vi "Configure Measurement Limits.vi"(7 "Upper Limit (2.0000000E+0)":dbl=2.0 format="%.7e", 8 "error in (no error)":errorcluster, 9 "Lower Limit (2.0000000E+0)":dbl=2.0 format="%.7e", 10 "Measurement Function (0: Voltage)":i32(ring) items=["Voltage", "Current", "Resistance"], 11 "VISA resource name":refnum<visa-resource-name>) -> (0 "error out":errorcluster, 3 "VISA resource name out":refnum<visa-resource-name>)   [LabVIEW 2019, in "Keithley 6517.lvlib"]
doc: "Configures the lower and upper limits for the measurement functions (Voltage, Current, Resistance and Charge).\n\nNote:\nThe specified measurement should be enabled from <b>Configure Measurement Function.vi</b>."
uses:
  Keithley 6517.lvlib
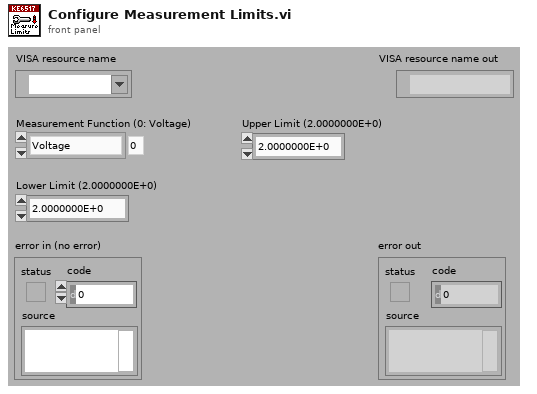
[diagram p1: front panel]
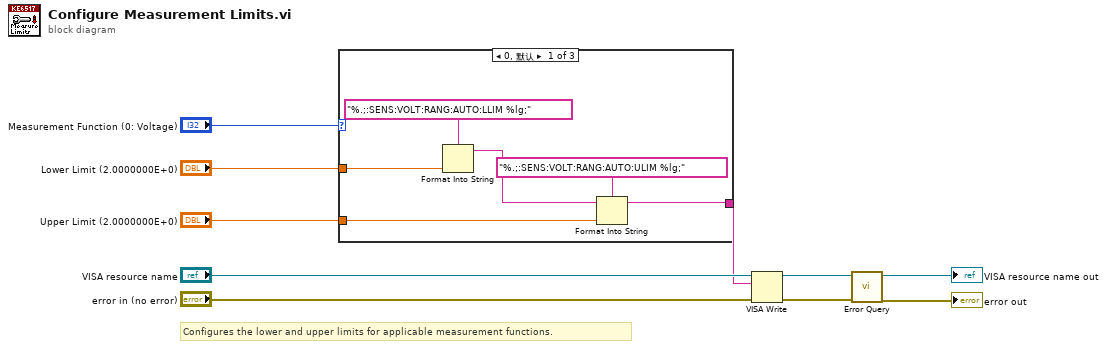
[diagram p0: block diagram]
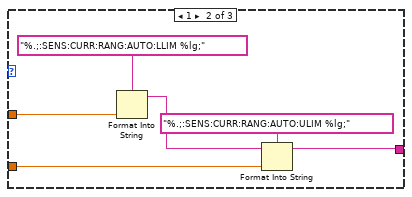
[diagram p2: hidden frame]
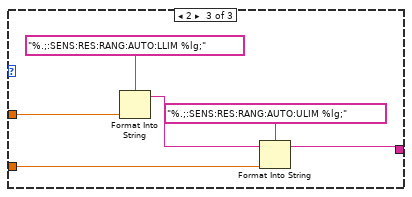
[diagram p3: hidden frame]
diagram:
  # "Configures the lower and upper limits for applicable measurement functions."
  n1 = case shown="0, 默认" "Measurement Function (0: Voltage)" {
    tunnel: "Lower Limit (2.0000000E+0)" -> [w13 w19 w25]
    tunnel: "Upper Limit (2.0000000E+0)" -> [w12 w18 w24]
    tunnel: [w11 w17 w23] -> w2
    frame 0, Default {
      n2 = Format Into String(format string="%.;:SENS:VOLT:RANG:AUTO:LLIM %lg;", w13) -> (resulting string=w15:string)  [unwired: 2 in, 1 out]
      n3 = Format Into String(format string="%.;:SENS:VOLT:RANG:AUTO:ULIM %lg;", initial string=w15, w12) -> (resulting string=w11:string)  [unwired: 1 in, 1 out]
    }
    frame 1 {
      n4 = Format Into String(format string="%.;:SENS:CURR:RANG:AUTO:LLIM %lg;", w19) -> (resulting string=w21:string)  [unwired: 2 in, 1 out]
      n5 = Format Into String(format string="%.;:SENS:CURR:RANG:AUTO:ULIM %lg;", initial string=w21, w18) -> (resulting string=w17:string)  [unwired: 1 in, 1 out]
    }
    frame 2 {
      n6 = Format Into String(format string="%.;:SENS:RES:RANG:AUTO:LLIM %lg;", w25) -> (resulting string=w28:string)  [unwired: 2 in, 1 out]
      n7 = Format Into String(format string="%.;:SENS:RES:RANG:AUTO:ULIM %lg;", initial string=w28, w24) -> (resulting string=w23:string)  [unwired: 1 in, 1 out]
    }
  }
  n8 = VISA Write(VISA resource name="VISA resource name", write buffer=w2, error in (no error)="error in (no error)") -> (VISA resource name out=w9:refnum<visa-resource-name>, error out=w8:errorcluster)  [unwired: 1 out]
  n9 = call "Error Query.vi"("error in (no error)"=w8, "VISA resource name"=w9) -> ("error out"=→"error out":errorcluster, "VISA resource name out"=→"VISA resource name out":refnum<visa-resource-name>)  [unwired: 6 in, 2 out]
